vi "CalibrateImageArray (SubVI).vi"(7 "error in (no error)":errorcluster, 10 "Image Array":T4[](array[typedef])) -> (0 "error out":errorcluster, 3 "Calibrated Image Array":T4[](array[typedef]))   [LabVIEW 2016]
uses:
  <vilib>/vision/Image Controls.llb/IMAQ Image.ctl
  <vilib>/vision/NI_Vision_Development_Module.lvlib
panel:
  in  "Pixel Distances":T1={"X Step"=3.5, "Y Step"=3.5, "Unit"=enum."Micrometer"} {"Y Step" format="%.2f"; "X Step" format="%.2f"}
  in  "Calibration Axis Info":T3={"Origin Pixel"={"X"=0.0, "Y"=0.0}, "Angle Relative to Horizontal (deg)"=0.0, "Axis Reference"=1} {"Axis Reference" items=["Direct", "Indirect"]}
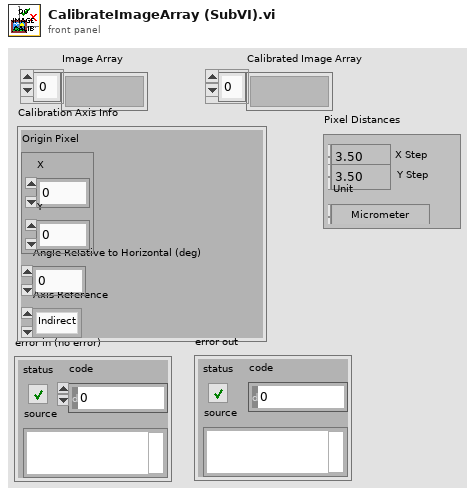
[diagram p1: front panel]
types:
  T1 = typedef "Simple Grid Descriptor" = cluster{"X Step":sgl, "Y Step":sgl, "Unit":T2}
  T2 = typedef "Image Unit" = enum32{"Undefined", "Angström", "Micrometer", "Millimeter", "Centimeter", "Meter", "Kilometer", "Microinch", "Inch", "Feet", "Nautical miles", "Standard miles", "Steps"}
  T3 = cluster{"Origin Pixel":cluster{"X":sgl, "Y":sgl}, "Angle Relative to Horizontal (deg)":sgl, "Axis Reference":u32}
  T4 = typedef "IMAQ Image.ctl" = refnum<image>
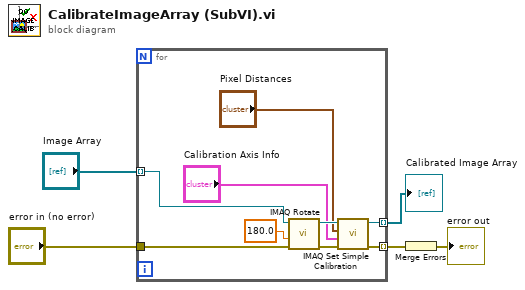
[diagram p0: block diagram]
diagram:
  n1 = for {
    tunnel: "Image Array" -> [w6] mode=indexing
    tunnel: "error in (no error)" -> [w14]
    tunnel: [w7] -> w5 mode=indexing
    tunnel: [w8] -> w2 mode=indexing
    n2 = call "IMAQ Rotate"("error in (no error)"=w14, "Angle (degrees)"=sgl 180.0, "Image Src"=w6) -> ("error out"=w9:errorcluster, "Image Dst Out"=w12:T4)  [unwired: 7 in]
    n3 = call "IMAQ Set Simple Calibration"("error in (no error)"=w9, "Calibration Axis Info"="Calibration Axis Info", "Grid Descriptor"="Pixel Distances", "Image"=w12) -> ("error out"=w8:errorcluster, "Calibrated Image"=w7:T4)  [unwired: 2 in, 4 out]
  }
  "Calibrated Image Array" <- w5
  n4 = Merge Errors(w2) -> (→"error out":errorcluster)
